vi "Add Rows (Variant).vi"(8 "error in (no error)":errorcluster, 9 "Data":variant[][](array[variant]), 11 "DataTable in":refnum<class "DataTable.lvclass">) -> (0 "error out":errorcluster, 3 "DataTable out":refnum<class "DataTable.lvclass">)   [LabVIEW 2013, in "DataGrid.lvlib" / "DataTable.lvclass"]
doc: "This allows any number of rows to be added to the datatable. The data must match the columns defined for the grid."
uses:
  DataTable.lvclass
  DataTable.lvclass/DataTable.ctl
  System.Data
  GridColumn/GridColumn.lvclass/GridColumn.ctl
  GridColumn/Read datatype.vi
  GridColumn/Read Params.vi
  GridColumn/Read Name.vi
  GridColumn/GridColumn.lvclass
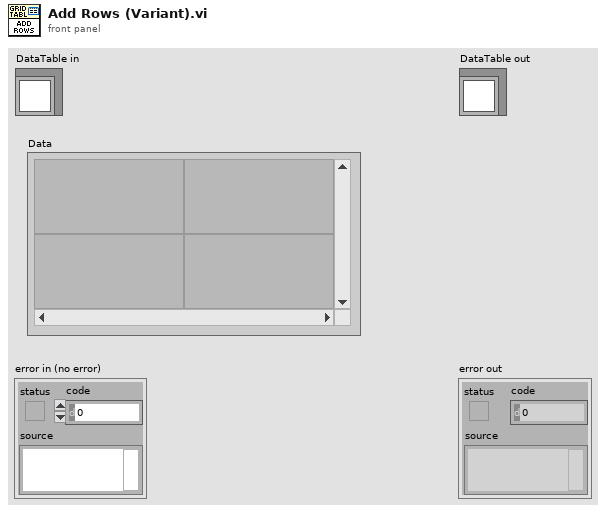
[diagram p1: front panel]
types:
  T1 = typedef "DataGrid.lvlib/GridColumn.lvclass/ColumnType.ctl" = enum16{"string", "image", "check", "numeric", "timestamp", "button", "combo", "link"}
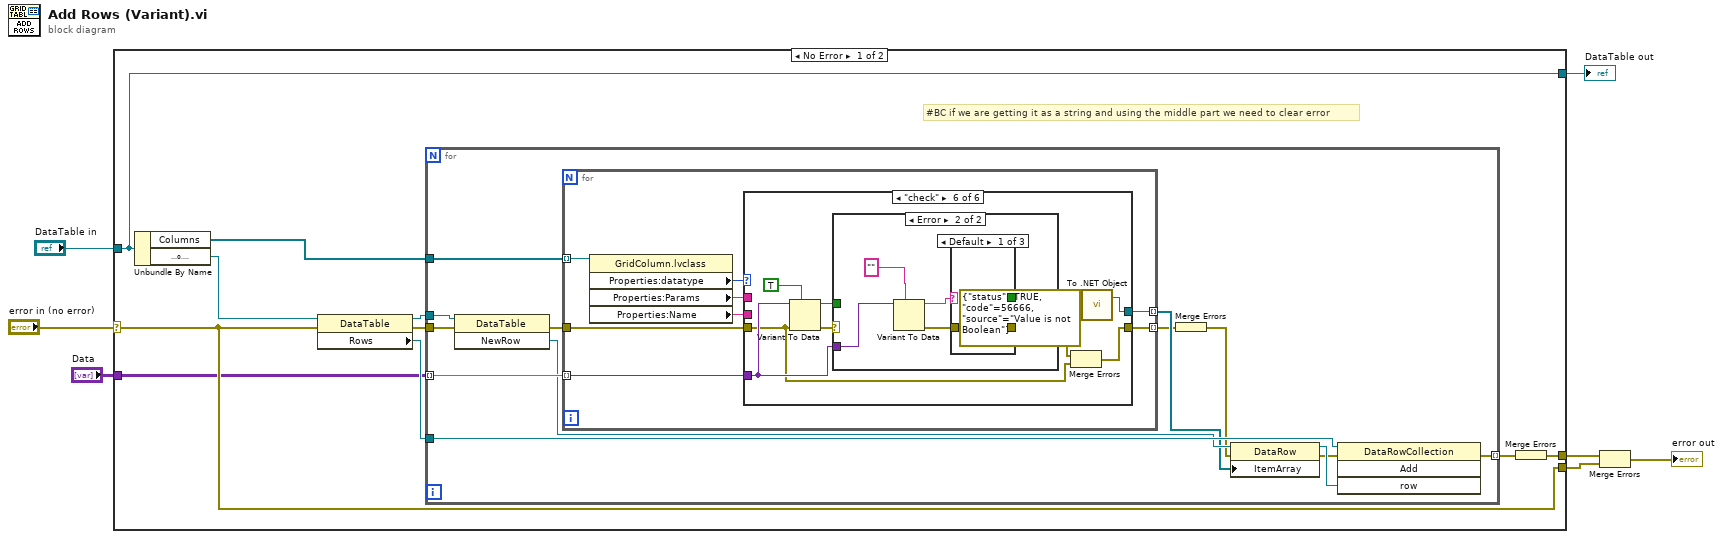
[diagram p0: block diagram]
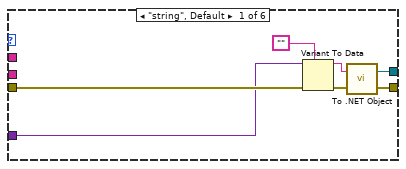
[diagram p2: hidden frame]
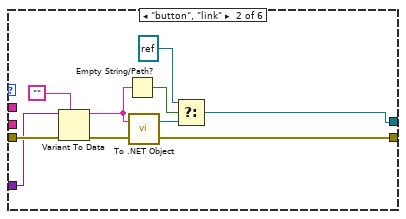
[diagram p3: hidden frame]
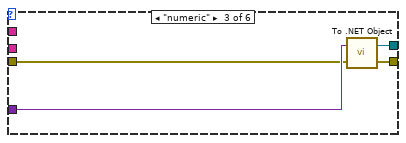
[diagram p4: hidden frame]
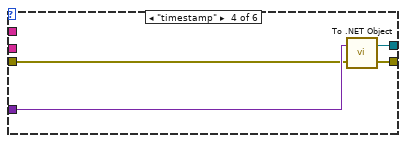
[diagram p5: hidden frame]
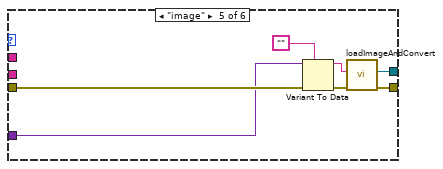
[diagram p6: hidden frame]
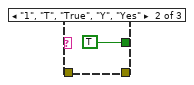
[diagram p8: hidden frame]
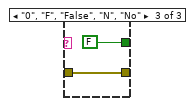
[diagram p9: hidden frame]
diagram:
  n1 = case shown="No Error" "error in (no error)" {
    selector: "error in (no error)" -> [w13 w93]
    tunnel: [w13 w93] -> w6
    tunnel: [w14 w92] -> w4
    tunnel: "DataTable in" -> [w14 w92]
    tunnel: "Data" -> [w12 _]
    tunnel: [w10 _] -> w1
    frame No Error {
      # "#BC if we are getting it as a string and using the middle part we need to clear error"
      n2 = Unbundle By Name(w14) -> ("Columns"=w9:refnum<class "GridColumn.lvclass">[], "DataTable"=w8:refnum<k24>)
      n3 = property class="DataTable"(reference=w8, error in=w13) -> (reference out=w11:refnum<k24>, error out=w17:errorcluster, "Rows"=w16:refnum<k24>)
      n4 = for {
        tunnel: w16 -> [w29]
        tunnel: w11 -> [w30]
        tunnel: [w28] -> w15 mode=indexing
        tunnel: w12 -> [w27] mode=indexing
        tunnel: w17 -> [w19]
        tunnel: w9 -> [w18]
        n5 = invoke class="DataTable" method="NewRow"(reference=w30, error in=w19) -> (error out=w26:errorcluster, "NewRow"=w25:refnum<k24>)  [unwired: 1 in, 1 out]
        n6 = for {
          tunnel: w27 -> [w38] mode=indexing
          tunnel: [w37] -> w23 mode=indexing
          tunnel: w26 -> [w36]
          tunnel: [w35] -> w22 mode=indexing
          tunnel: w18 -> [w34] mode=indexing
          n7 = property class="GridColumn.lvclass"(reference=w34) -> ("Properties:datatype"=w33:T1, "Properties:Params"=w32:string, "Properties:Name"=w31:string)  [unwired: 1 in, 2 out]
          n8 = case shown="\"check\"" w33 {
            tunnel: w38 -> [w42 w52 w57 w61 w66 w74]
            tunnel: [w41 w49 w58 w62 w70 w79] -> w37
            tunnel: w36 -> [w45 w55 w56 w60 w68 w72]
            tunnel: [w43 w53 w59 w63 w69 w71] -> w35
            tunnel: w32 -> [_ _ _ _ _ _]
            tunnel: w31 -> [_ _ _ _ _ _]
            frame "string", Default {
              n9 = Variant To Data(error in=w45, type="", Variant=w42) -> (data=w40:string, error out=w44:errorcluster)
              n10 = call <vilib>:"To .NET Object.vi"("error in (no error)"=w44, "anything"=w40) -> ("error out"=w43:errorcluster, ".NET object"=w41:refnum<k24>)
            }
            frame "button", "link" {
              n11 = Variant To Data(error in=w55, type="", Variant=w52) -> (data=w46:string, error out=w54:errorcluster)
              n12 = Empty String/Path?(string/path=w46) -> (empty?=w51:bool)
              n13 = call <vilib>:"To .NET Object.vi"("error in (no error)"=w54, "anything"=w46) -> ("error out"=w53:errorcluster, ".NET object"=w50:refnum<k24>)
              n14 = Select(t=refnum<k24> refnum, s=w51, f=w50) -> (s? t:f=w49:refnum<k24>)
            }
            frame "numeric" {
              n15 = call <vilib>:"To .NET Object.vi"("error in (no error)"=w56, "anything"=w57) -> ("error out"=w59:errorcluster, ".NET object"=w58:refnum<k24>)
            }
            frame "timestamp" {
              n16 = call <vilib>:"To .NET Object.vi"("error in (no error)"=w60, "anything"=w61) -> ("error out"=w63:errorcluster, ".NET object"=w62:refnum<k24>)
            }
            frame "image" {
              n17 = Variant To Data(error in=w68, type="", Variant=w66) -> (data=w64:string, error out=w67:errorcluster)
              n18 = call "loadImageAndConvert.vi"("error in (no error)"=w67, "name or relative path"=w64) -> ("error out"=w69:errorcluster, ".NET object"=w70:refnum<k24>)  [unwired: 8 in]
            }
            frame "check" {
              n19 = Variant To Data(error in=w72, type=TRUE, Variant=w74) -> (data=w75:bool, error out=w76:errorcluster)
              n20 = case shown="Error" w76 {
                selector: w76 -> [w81 _]
                tunnel: [w80 w87] -> w78
                tunnel: [w81 w82] -> w73
                tunnel: w75 -> [w80 _]
                tunnel: w74 -> [_ w85]
                frame No Error {
                }
                frame Error {
                  n21 = Variant To Data(type="", Variant=w85) -> (data=w86:string, error out=w83:errorcluster)  [unwired: 1 in]
                  n22 = case shown="Default" w86 {
                    tunnel: [_ TRUE FALSE] -> w87
                    tunnel: w83 -> [_ _ w90]
                    tunnel: [errorcluster {"status"=TRUE, "code"=56666, "source"="Value is not Boolean"} ("error out") _ w90] -> w82
                    frame Default {
                    }
                    frame "1", "T", "True", "Y", "Yes" {
                    }
                    frame "0", "F", "False", "N", "No" {
                    }
                  }
                }
              }
              n23 = Merge Errors(w73, w72) -> (w71:errorcluster)
              n24 = call <vilib>:"To .NET Object.vi"("anything"=w78) -> (".NET object"=w79:refnum<k24>)  [unwired: 1 in, 1 out]
            }
          }
        }
        n25 = Merge Errors(w22) -> (w21:errorcluster)
        n26 = property class="DataRow"(reference=w25, error in=w21, "ItemArray"=w23) -> (reference out=w24:refnum<k24>, error out=w20:errorcluster)
        n27 = invoke class="DataRowCollection" method="Add"(reference=w29, error in=w20, "row"=w24) -> (error out=w28:errorcluster)  [unwired: 1 in, 3 out]
      }
      n28 = Merge Errors(w15) -> (w10:errorcluster)
    }
    frame Error {
    }
  }
  "DataTable out" <- w4
  n29 = Merge Errors(w1, w6) -> (→"error out":errorcluster)
